vi "basic - Transmit UDP Queuing.vi"() -> ()   [LabVIEW 2020]
uses:
  _controls/comm_computedMAC-IP.ctl
  _controls/comm_udp_tx.ctl
  _controls/comm_config_vl_tx.ctl
  _polimorphicInstances/session/Fdx Create Session (Tx-UDP Port-Oriented).vi
  bsp/AFDX_Transmit/Fdx Create Tx VL.vi
  _polimorphicInstances/udpPort/Fdx Create UDP Port (TX-CommPort).vi
  _polimorphicInstances/control/Fdx Start (Tx).vi
  _polimorphicInstances/control/Fdx Stop (Tx).vi
  _polimorphicInstances/session/Fdx Close Session (Port).vi
  AIM664LV.lvlib
panel:
  out "Duplicated":bool
  in  "VL Config":T1={"VlId"=60, "NumOfSubVl"=2, "rate mS (128)"=128.0, "domainID"=1, "sideID"=1, "locationID"=1, "interfaceID"=1, "NetSelect"=3, "Skew"=0, "MaxFrameLength"=1000, "FrameBufferSize"=0} {"NetSelect" items=["FDX_TX_FRAME_DLY_A"=0, "FDX_TX_FRAME_DLY_B"=1, "FDX_TX_FRAME_BOTH "=3, "FDX_TX_FRAME_ONLY_A"=4, "FDX_TX_FRAME_ONLY_B "=5]; "interfaceID" format="%.0b"}
  in  "CommPort Config":T2[](array[typedef])=[{"PortType"=enum."FDX_UDP_QUEUING", "partitionID"=1, "SubVlId"=1, "UdpSrcPort"=1, "UdpDstPort"=1, "SampleRateMs"=128.0, "UdpNumBufMessages"=0, "UdpMaxMessageSize"=1000}, {"PortType"=enum."FDX_UDP_QUEUING", "partitionID"=1, "SubVlId"=2, "UdpSrcPort"=2, "UdpDstPort"=2, "SampleRateMs"=128.0, "UdpNumBufMessages"=0, "UdpMaxMessageSize"=1000}]
  in  "millisecond multiple":u32=128
  in  "PortMap":u32
  out "IndexCycleCount":u32[](array[numeric])
  out "MsgCount":u32[](array[numeric])
  out "CurrentIndex":u32[](array[numeric])
  out "BytesWritten":u32[](array[numeric])
  in  "port":u32
  in  "board":u32
  out "current time":timestamp=timestamp(3677762637.591913 s since 1904-01-01)
  out "current irig time":T3={"SignOut"=40, "DayOut"=1, "HourOut"=1, "MinOut"=28, "SecondOut"=39, "MilliSecOut"=539, "MicroSecOut"=300, "NanoSecOut"=0, "InfoOut"=0, "Mode"=3}
  out "CommPort Addresses":T4[](array[typedef]) {"MACsrc" format="%.0x"}
  in  "Data to be sent":u8[](array[numeric])=[255, 255, 255, 255, 255, 255, 255, 255, 255, 255, 255, 255, 255, 255, 255, 255, 255, 255, 255, 255, 255, 255, 255, 255, 255, 255, 255, 255, 255, 255, 255, 255, 255, 255, 255, 255, 255, 255, 255, 255, 255, 255, 255, 255, 255, 255, 255, 255, 255, 255, 255, 255, 255, 255, 255, 255, 255, 255, 255, 255, 255, 255, 255, 255, 255, 255, 255, 255, 255, 255, 255, 255, 255, 255, 255, 255, 255, 255, 255, 255, 255, 255, 255, 255, 255, 255, 255, 255, 255, 255, 255, 255, 255, 255, 255, 255, 255, 255, 255, 170] format="%.0x"
  in  "stop":bool
  out "PortInitOut":T5={"PortConfig"=0, "PortUsed"=1, "GlobalMemFree"=0, "SharedMemFree"=0} {"PortConfig" items=["FDX_SINGLE", "FDX_REDUNDANT"]}
  out "error out":errorcluster
  # "ARINC 664 - Transmit UDP - Queuing Port"
  # "Overview: Setup the board to transmit package as UDP using Queue format. \n\nRequirement: One AIM ARINC-664 board with installed AIM ARINC 664 BSP.\nRestrictions: None.\nInstruction:\n1. Select the Board ID (0 if you have only one board in your system) and the port number. If you want to validate between two ports in one device, you can use tx board and Rx Boardd\n2. Run the VI.\n3. See the result in Current IRIG Time"
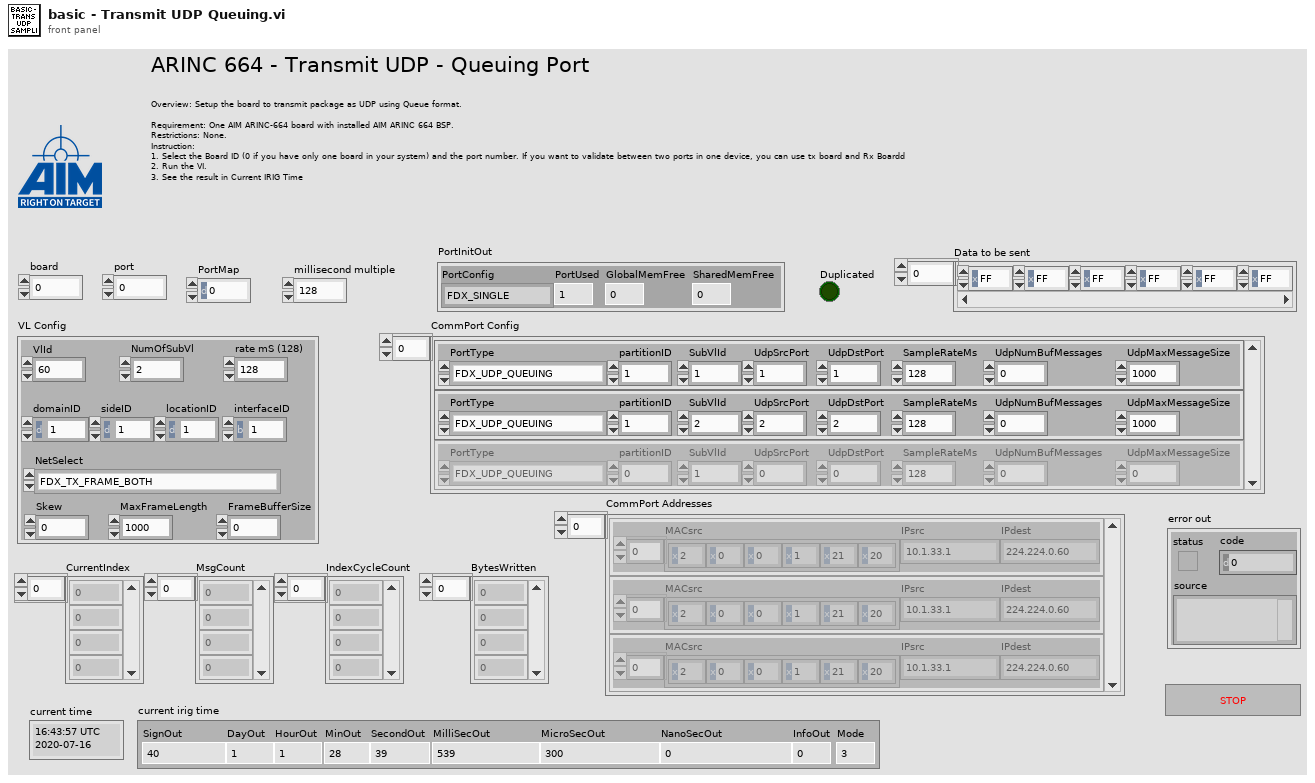
[diagram p1: front panel]
types:
  T1 = typedef "AIM664LV.lvlib/comm_config_vl_tx.ctl" = cluster{"VlId":u16, "NumOfSubVl":u16, "rate mS (128)":dbl, "domainID":u8, "sideID":u8, "locationID":u8, "interfaceID":u8, "NetSelect":u32, "Skew":u32, "MaxFrameLength":u32, "FrameBufferSize":u32}
  T2 = typedef "AIM664LV.lvlib/comm_udp_tx.ctl" = cluster{"PortType":enum16{"FDX_UDP_SAMPLING", "FDX_UDP_QUEUING"}, "partitionID":u8, "SubVlId":u8, "UdpSrcPort":u16, "UdpDstPort":u16, "SampleRateMs":dbl, "UdpNumBufMessages":u32, "UdpMaxMessageSize":u32}
  T3 = cluster{"SignOut":i32, "DayOut":u32, "HourOut":u32, "MinOut":u32, "SecondOut":u32, "MilliSecOut":u32, "MicroSecOut":u32, "NanoSecOut":u32, "InfoOut":u32, "Mode":u32}
  T4 = typedef "AIM664LV.lvlib/comm_computedMAC-IP.ctl" = cluster{"MACsrc":u8[], "IPsrc":string, "IPdest":string}
  T5 = cluster{"PortConfig":u32, "PortUsed":u32, "GlobalMemFree":u32, "SharedMemFree":u32}
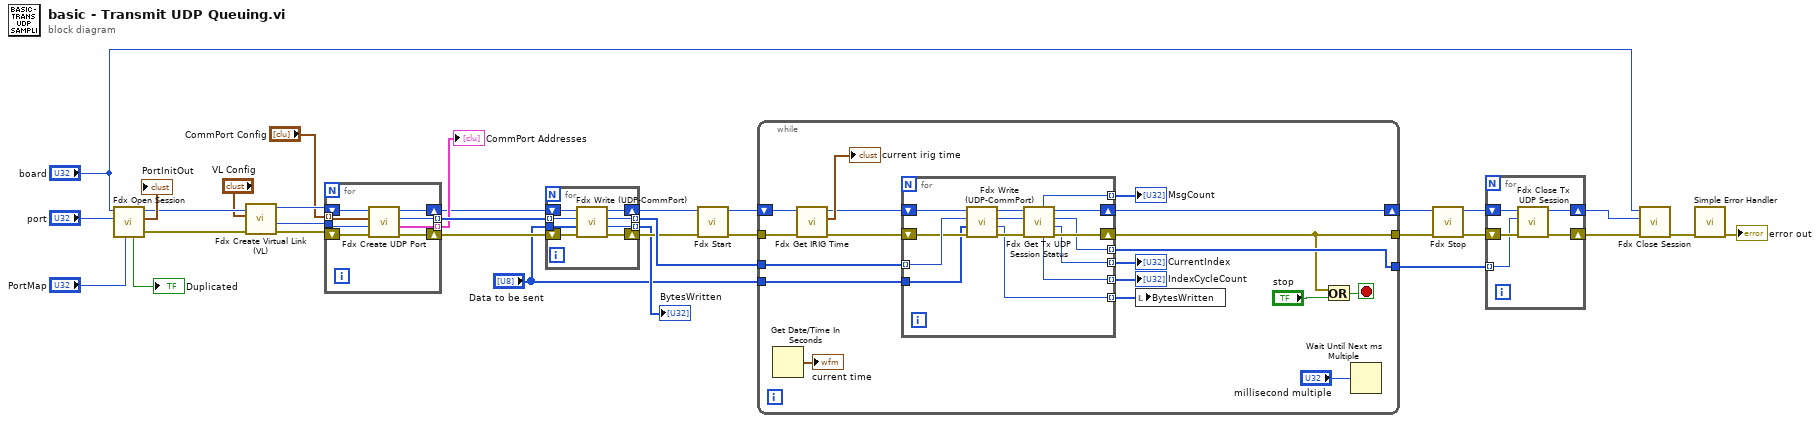
[diagram p0: block diagram]
diagram:
  n1 = call-poly "Fdx Open Session.vi"("PortMap"="PortMap", "port"="port", "board"="board") -> ("error out"=w15:errorcluster, "PortInitOut"=→"PortInitOut":T5, "port handle out"=w16:u32, "Duplicated"=→"Duplicated":bool)  [unwired: 4 in, 1 out]
  n2 = call-poly "Fdx Create Virtual Link (VL).vi"("error in (no error)"=w15, "VL Config"="VL Config", "InstrumentHandle in"=w16) -> ("error out"=w13:errorcluster, "VlId"=w12:u16, "InstrumentHandle out"=w14:u32)  [unwired: 6 in]
  n3 = for {
    tunnel: [w39] -> w31 mode=indexing
    tunnel: [w36] -> w28 mode=indexing
    shift-right: [w35] -> w7
    shift-left: w14 -> [w40]
    shift-right: [w38] -> w29
    shift-left: w13 -> [w37]
    tunnel: w12 -> [w34]
    tunnel: "CommPort Config" -> [w33] mode=indexing
    n4 = call-poly "Fdx Create UDP Port.vi"("error in"=w37, "VlId"=w34, "CommPort Config"=w33, "port handle in"=w40) -> ("error out"=w38:errorcluster, "computedAddresses"=w36:T4, "commPort handle out"=w39:u32, "port handle out"=w35:u32)  [unwired: 4 in]
  }
  "CommPort Addresses" <- w28
  n5 = for {
    tunnel: "Data to be sent" -> [w44]
    tunnel: [w46] -> w18 mode=indexing
    shift-right: [w47] -> w26
    shift-left: w29 -> [w48]
    tunnel: w31 -> [w45] mode=indexing
    tunnel: [w41] -> w30 mode=indexing
    shift-right: [w42] -> w6
    shift-left: w7 -> [w43]
    n6 = call "Fdx Write (UDP-CommPort).vi"("error in (no error)"=w48, "Data"=w44, "UdpHandle in"=w45, "InstrumentHandle_port in"=w43) -> ("error out"=w47:errorcluster, "BytesWritten"=w46:u32, "UdpHandle out"=w41:u32, "InstrumentHandle_port out"=w42:u32)  [unwired: 4 in]
  }
  "BytesWritten" <- w18
  n7 = call-poly "Fdx Start.vi"("error in (no error)"=w26, "InstrumentHandle_port in"=w6) -> ("error out"=w25:errorcluster, "InstrumentHandle_port out"=w24:u32)  [unwired: 8 in]
  n8 = while {
    tunnel: w25 -> [w62]
    tunnel: w30 -> [w54]
    tunnel: [w59] -> w21
    tunnel: [w58] -> w22
    shift-right: [w50] -> w27
    shift-left: w24 -> [w63]
    tunnel: "Data to be sent" -> [w49]
    stop <- w65 stop-if-true
    n9 = Get Date/Time In Seconds() -> (seconds since 1Jan1904=→"current time":timestamp)
    n10 = call "Fdx Get IRIG Time.vi"("error in (no error)"=w62, "InstrumentHandle_board in"=w63) -> ("error out"=w53:errorcluster, "Curent Irig Time"=→"current irig time":T3, "InstrumentHandle_board out"=w51:u32)  [unwired: 7 in]
    n11 = for {
      tunnel: [w68] -> w59 mode=indexing
      tunnel: [w79] -> w57 mode=indexing
      tunnel: [w69] -> w56 mode=indexing
      tunnel: [w78] -> w55 mode=indexing
      tunnel: w54 -> [w77] mode=indexing
      tunnel: [w73] -> w52 mode=indexing
      tunnel: w49 -> [w72]
      shift-right: [w80] -> w58
      shift-left: w53 -> [w76]
      shift-right: [w67] -> w50
      shift-left: w51 -> [w71]
      n12 = call "Fdx Write (UDP-CommPort).vi"("error in (no error)"=w76, "Data"=w72, "UdpHandle in"=w77, "InstrumentHandle_port in"=w71) -> ("error out"=w75:errorcluster, "BytesWritten"=w73:u32, "UdpHandle out"=w70:u32, "InstrumentHandle_port out"=w74:u32)  [unwired: 4 in]
      n13 = call "Fdx Get Tx UDP Session Status.vi"("error in (no error)"=w75, "UdpHandle in"=w70, "InstrumentHandle_port in"=w74) -> ("error out"=w80:errorcluster, "CurrentIndex"=w79:u32, "UdpHandle out"=w68:u32, "InstrumentHandle_port out"=w67:u32, "IndexCycleCount"=w78:u32, "MsgCount"=w69:u32)  [unwired: 3 in]
    }
    "CurrentIndex" <- w57
    "MsgCount" <- w56
    "IndexCycleCount" <- w55
    n14 = local write "BytesWritten"(w52) -> ()
    n15 = Or(x=w58, y="stop") -> (x .or. y?=w65:bool)
    n16 = Wait Until Next ms Multiple(millisecond multiple="millisecond multiple") -> ()  [unwired: 1 out]
  }
  n17 = call-poly "Fdx Stop.vi"("error in (no error)"=w22, "InstrumentHandle_port in"=w27) -> ("error out"=w20:errorcluster, "InstrumentHandle_port out"=w5:u32)  [unwired: 8 in]
  n18 = for {
    tunnel: w21 -> [w83] mode=indexing
    shift-right: [w84] -> w19
    shift-left: w20 -> [w85]
    shift-right: [w81] -> w4
    shift-left: w5 -> [w82]
    n19 = call "Fdx Close Tx UDP Session.vi"("error in (no error)"=w85, "UdpHandle in"=w83, "InstrumentHandle_port in"=w82) -> ("error out"=w84:errorcluster, "InstrumentHandle_port out"=w81:u32)  [unwired: 7 in]
  }
  n20 = call-poly "Fdx Close Session.vi"("error in"=w19, "InstrumentHandle_port in"=w4, "InstrumentHandle_board in"="board") -> ("error out"=w1:errorcluster)  [unwired: 8 in]
  n21 = call <vilib>:"Simple Error Handler.vi"("error in (no error)"=w1) -> ("error out"=→"error out":errorcluster)  [unwired: 4 in, 4 out]
